vi "Copy Errors to Built Directory.vi"(11 "Arguments":string[](array[string])) -> (2 "Output/Failure Message":string, 3 "Exit Code":i32)   [LabVIEW 2027]
panel:
  out "error out":errorcluster
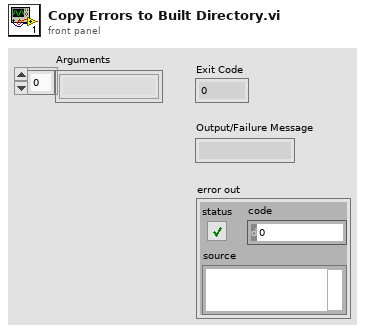
[diagram p1: front panel]
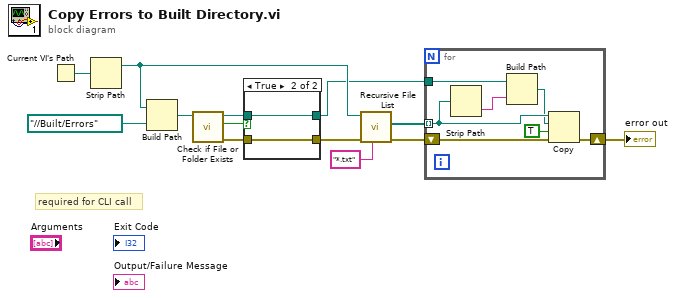
[diagram p0: block diagram]
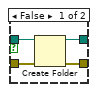
[diagram p2: hidden frame]
diagram:
  # "required for CLI call"
  n1 = Current VI's Path() -> (path=w13:path)
  n2 = Strip Path(path=w13) -> (stripped path=w7:path)  [unwired: 1 out]
  n3 = Build Path(base path=w7, name or relative path=path "../../Built/Errors" ("stripped path")) -> (appended path=w6:path)
  n4 = call <vilib>:"Check if File or Folder Exists.vi"("path"=w6) -> ("error out"=w4:errorcluster, "file or folder exists?"=w5:bool, "dup path"=w3:path)  [unwired: 8 in]
  n5 = case shown="True" w5 {
    tunnel: w4 -> [w16 w19]
    tunnel: w3 -> [w17 w18]
    tunnel: [w15 w19] -> w2
    tunnel: [w14 w18] -> w1
    frame False {
      n6 = Create Folder(path (use dialog)=w17, error in=w16) -> (created path=w14:path, error out=w15:errorcluster)  [unwired: 1 in, 1 out]
    }
    frame True {
    }
  }
  n7 = call <vilib>:"Recursive File List.vi"("pattern"="*.txt", "error in (no error)"=w2, "Folder Path"=w7) -> ("error out"=w10:errorcluster, "All Files in Dir"=w11:path[])  [unwired: 4 in, 3 out]
  n8 = for {
    tunnel: w11 -> [w24] mode=indexing
    tunnel: w1 -> [w25]
    shift-right: [w20] -> w8
    shift-left: w10 -> [w26]
    n9 = Strip Path(path=w24) -> (name=w23:string)  [unwired: 1 out]
    n10 = Build Path(base path=w25, name or relative path=w23) -> (appended path=w22:path)
    n11 = Copy(8:w26, 9:TRUE ("overwrite (F)"), 10:w22, 11:w24) -> (0:w20:errorcluster)  [unwired: 1 in, 2 out]
  }
  "error out" <- w8
